vi "LDA_IP.vi"() -> (15 "error out":errorcluster)   [LabVIEW 2012]
uses:
  Globals/Meas_global.vi
  Globals/LDA_meas_global_1.vi
  Globals/LDA_meas_global_2.vi
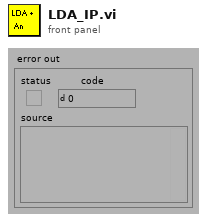
[diagram p1: front panel]
types:
  T1 = typedef "Ch_and_Spans.ctl" = cluster{"high limit (10V)":sgl, "low limit (-10V)":sgl, "Ch No":i16, "Var name":string, "Use Latest Calib":bool}
  T2 = typedef "LDA_Setup.ctl" = cluster{"dimensions":enum16{"1D", "2D"}, "Analogue Freq Multiplier":dbl}
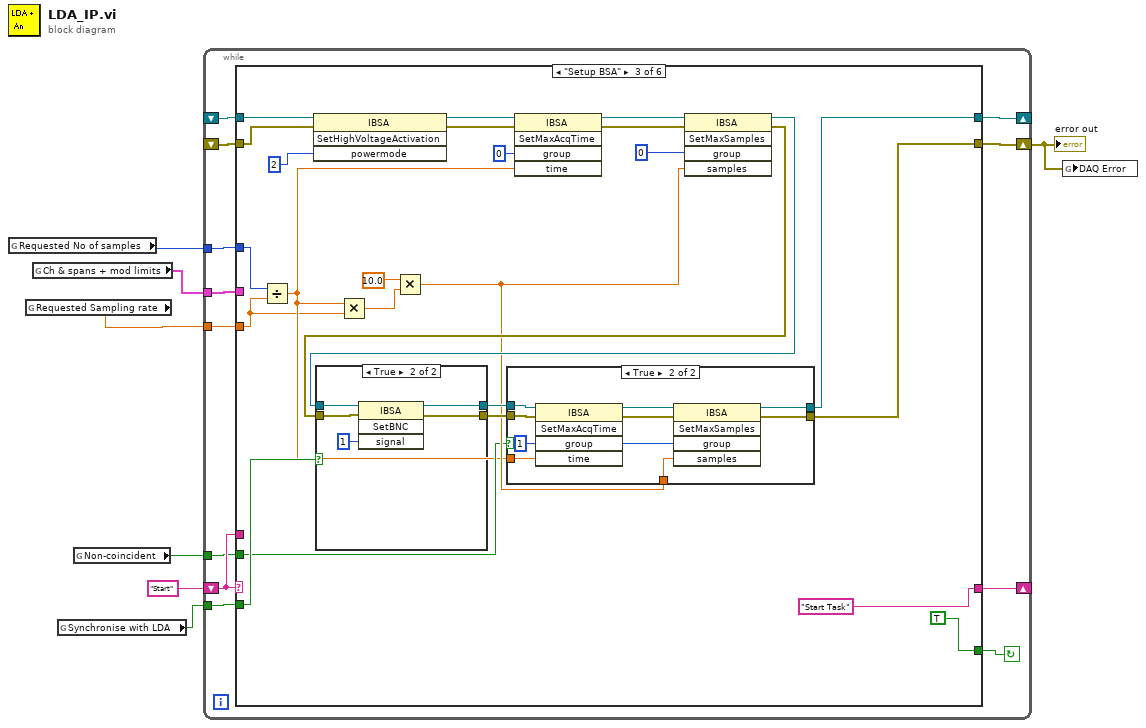
[diagram p0: block diagram]
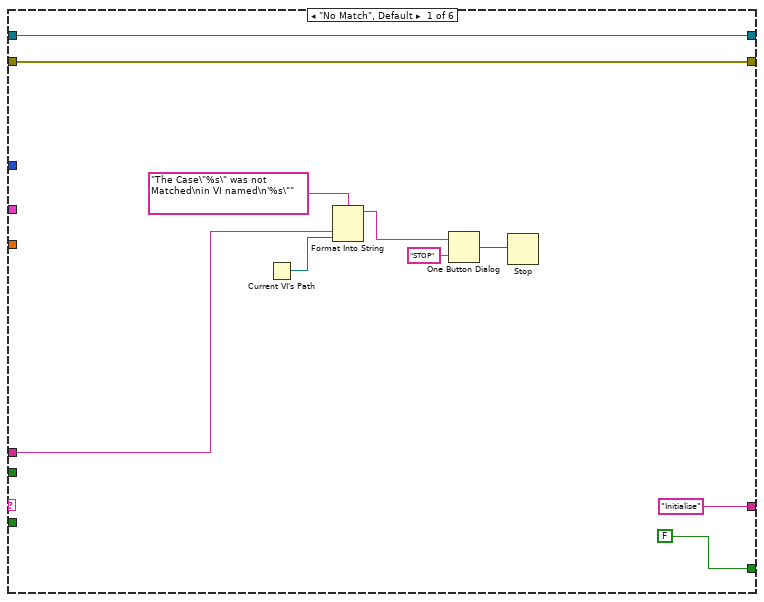
[diagram p2: hidden frame]
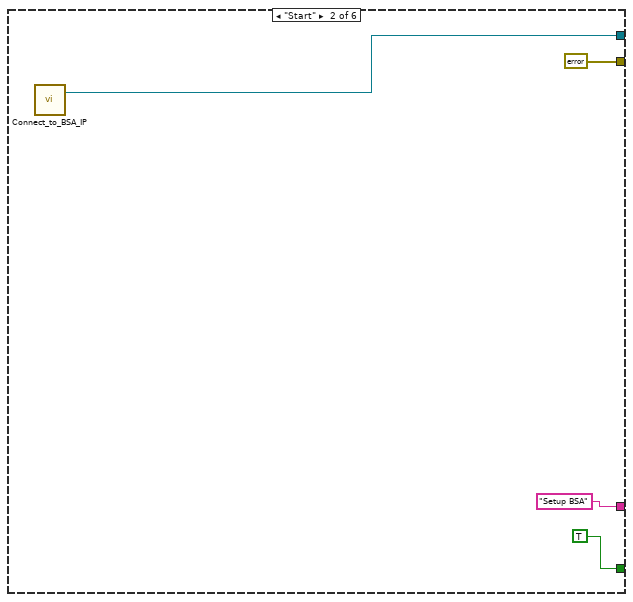
[diagram p3: hidden frame]
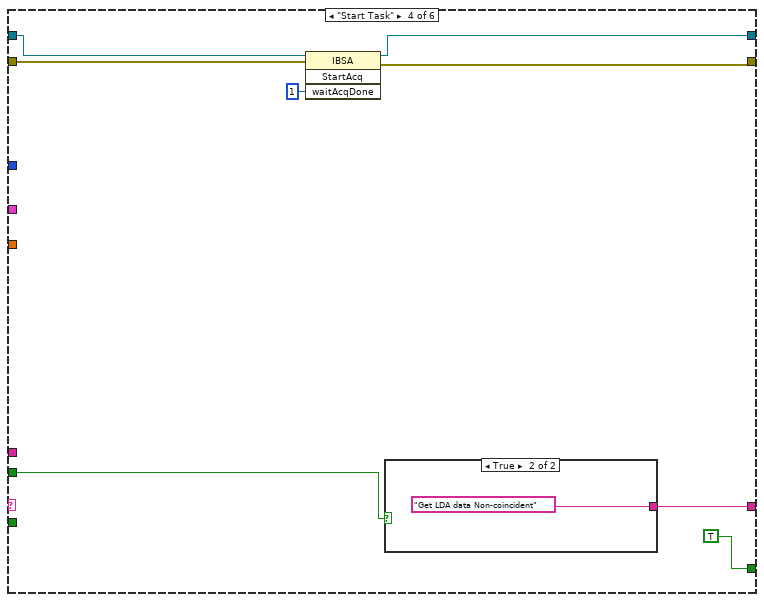
[diagram p6: hidden frame]
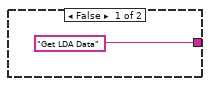
[diagram p7: hidden frame]
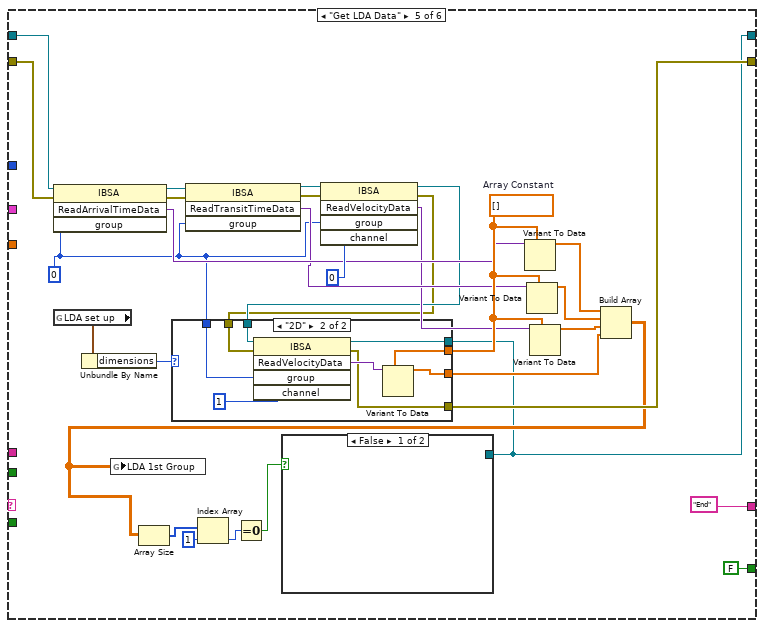
[diagram p8: hidden frame]
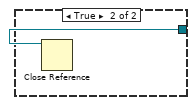
[diagram p9: hidden frame]
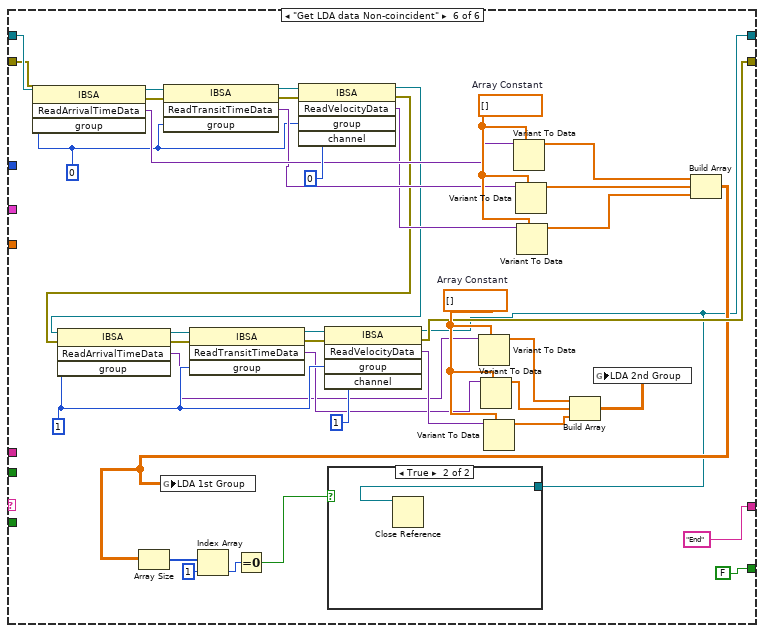
[diagram p11: hidden frame]
diagram:
  n1 = global read "Meas_global.vi" "Requested No of samples"() -> (w2:i32)
  n2 = global read "Meas_global.vi" "Requested Sampling rate"() -> (w3:dbl)
  n3 = global read "Meas_global.vi" "Ch & spans + mod limits"() -> (w4:T1[])
  n4 = global read "Meas_global.vi" "Synchronise with LDA"() -> (w6:bool)
  n5 = global read "LDA_meas_global_1.vi" "Non-coincident"() -> (w5:bool)
  n6 = while {
    shift-left: "Start" -> [w17]
    shift-right: [w18] -> _
    shift-right: [w13] -> w1
    shift-left: _ -> [w16]
    tunnel: w2 -> [w15]
    tunnel: w4 -> [w14]
    tunnel: w3 -> [w12]
    shift-right: [w10] -> _
    shift-left: _ -> [w11]
    tunnel: w6 -> [w9]
    tunnel: w5 -> [w8]
    stop <- w19 continue-if-true
    n7 = case shown="\"Setup BSA\"" w17 {
      tunnel: [FALSE TRUE TRUE TRUE FALSE FALSE] -> w19
      tunnel: ["Initialise" "Setup BSA" "Start Task" w79 "End" "End"] -> w18
      tunnel: w17 -> [w24 _ _ _ _ _]
      tunnel: [w21 errorcluster {"status"=FALSE, "code"=0, "source"=""} ("error out") w40 w83 w98 w139] -> w13
      tunnel: w16 -> [w21 _ w49 w80 w92 w137]
      tunnel: w15 -> [_ _ w50 _ _ _]
      tunnel: w14 -> [_ _ _ _ _ _]
      tunnel: w12 -> [_ _ w35 _ _ _]
      tunnel: w11 -> [w20 _ w51 w82 w102 w138]
      tunnel: [w20 w30 w42 w81 w88 w130] -> w10
      tunnel: w9 -> [_ _ w44 _ _ _]
      tunnel: w8 -> [_ _ w38 w78 _ _]
      frame "No Match", Default {
        n8 = Current VI's Path() -> (path=w23:path)
        n9 = Format Into String(format string="The Case\"%s\" was not Matched\nin VI named\n'%s\"" ("Format String"), w24, w23) -> (resulting string=w27:string)  [unwired: 2 in, 1 out]
        n10 = One Button Dialog(message=w27, button name ("OK")="STOP") -> (true=w25:bool)
        n11 = Stop(stop? (T)=w25) -> ()
      }
      frame "Start" {
        n12 = call "Connect_to_BSA_IP.vi"() -> ("BSA"=w30:refnum<k7>)  [unwired: 3 out]
      }
      frame "Setup BSA" {
        n13 = Divide(x=w50, y=w35) -> (x/y=w36:dbl)
        n14 = invoke class="IBSA" method="SetHighVoltageActivation"(reference=w51, error in=w49, "powermode"=2) -> (reference out=w56:refnum<k7>, error out=w58:errorcluster)  [unwired: 1 in, 2 out]
        n15 = Multiply(x=w36, y=w35) -> (x*y=w34:dbl)
        n16 = Multiply(x=10.0 ("y"), y=w34) -> (x*y=w39:dbl)
        n17 = invoke class="IBSA" method="SetMaxAcqTime"(reference=w56, error in=w58, "group"=0, "time"=w36) -> (reference out=w57:refnum<k7>, error out=w55:errorcluster)  [unwired: 1 in, 3 out]
        n18 = invoke class="IBSA" method="SetMaxSamples"(reference=w57, error in=w55, "group"=0, "samples"=w39) -> (reference out=w46:refnum<k7>, error out=w45:errorcluster)  [unwired: 1 in, 3 out]
        n19 = case shown="True" w44 {
          tunnel: w46 -> [w70 w75]
          tunnel: w45 -> [w71 w74]
          tunnel: [w70 w73] -> w43
          tunnel: [w71 w72] -> w41
          frame False {
          }
          frame True {
            n20 = invoke class="IBSA" method="SetBNC"(reference=w75, error in=w74, "signal"=1) -> (reference out=w73:refnum<k7>, error out=w72:errorcluster)  [unwired: 1 in, 2 out]
          }
        }
        n21 = case shown="True" w38 {
          tunnel: w43 -> [w60 w67]
          tunnel: [w60 w65] -> w42
          tunnel: w41 -> [w59 w64]
          tunnel: [w59 w63] -> w40
          tunnel: w36 -> [_ w62]
          tunnel: w39 -> [_ w61]
          frame False {
          }
          frame True {
            w68 = 1 ("group")
            n22 = invoke class="IBSA" method="SetMaxAcqTime"(reference=w67, error in=w64, "group"=w68, "time"=w62) -> (reference out=w66:refnum<k7>, error out=w69:errorcluster)  [unwired: 1 in, 3 out]
            n23 = invoke class="IBSA" method="SetMaxSamples"(reference=w66, error in=w69, "group"=w68, "samples"=w61) -> (reference out=w65:refnum<k7>, error out=w63:errorcluster)  [unwired: 1 in, 3 out]
          }
        }
      }
      frame "Start Task" {
        n24 = invoke class="IBSA" method="StartAcq"(reference=w82, error in=w80, "waitAcqDone"=1) -> (reference out=w81:refnum<k7>, error out=w83:errorcluster)  [unwired: 1 in, 2 out]
        n25 = case shown="True" w78 {
          tunnel: ["Get LDA Data" "Get LDA data Non-coincident"] -> w79
          frame False {
          }
          frame True {
          }
        }
      }
      frame "Get LDA Data" {
        w110 = dbl[] []  # Array Constant
        w99 = 0 ("group")
        n26 = invoke class="IBSA" method="ReadArrivalTimeData"(reference=w102, error in=w92, "group"=w99) -> (reference out=w115:refnum<k7>, error out=w114:errorcluster, "ReadArrivalTimeData"=w109:variant)  [unwired: 1 in, 1 out]
        n27 = global read "Meas_global.vi" "LDA set up"() -> (w91:T2)
        n28 = Unbundle By Name(w91) -> ("dimensions"=w90:enum16{"1D", "2D"})
        n29 = invoke class="IBSA" method="ReadTransitTimeData"(reference=w115, error in=w114, "group"=w99) -> (reference out=w113:refnum<k7>, error out=w112:errorcluster, "ReadTransitTimeData"=w108:variant)  [unwired: 1 in, 1 out]
        n30 = invoke class="IBSA" method="ReadVelocityData"(reference=w113, error in=w112, "group"=w99, "channel"=0) -> (reference out=w101:refnum<k7>, error out=w100:errorcluster, "ReadVelocityData"=w107:variant)  [unwired: 1 in, 2 out]
        n31 = case shown="\"2D\"" w90 {
          tunnel: w110 -> [w118 w127]
          tunnel: [w118 w125] -> w103
          tunnel: [w119 w124] -> w88
          tunnel: w101 -> [w119 w123]
          tunnel: w100 -> [w117 w122]
          tunnel: w99 -> [_ w121]
          tunnel: [w117 w120] -> w98
          frame "1D" {
          }
          frame "2D" {
            n32 = invoke class="IBSA" method="ReadVelocityData"(reference=w123, error in=w122, "group"=w121, "channel"=1) -> (reference out=w124:refnum<k7>, error out=w120:errorcluster, "ReadVelocityData"=w126:variant)  [unwired: 1 in, 2 out]
            n33 = Variant To Data(type=w127, Variant=w126) -> (data=w125:dbl[])  [unwired: 1 in, 1 out]
          }
        }
        n34 = Variant To Data(type=w110, Variant=w109) -> (data=w106:dbl[])  [unwired: 1 in, 1 out]
        n35 = Variant To Data(type=w110, Variant=w108) -> (data=w105:dbl[])  [unwired: 1 in, 1 out]
        n36 = Variant To Data(type=w110, Variant=w107) -> (data=w104:dbl[])  [unwired: 1 in, 1 out]
        n37 = Build Array(w106, w105, w104, w103) -> (w93:dbl[][])
        n38 = global write "LDA_meas_global_2.vi" "LDA 1st Group"(w93) -> ()
        n39 = Array Size(array=w93) -> (size(s)=w97:i32[])
        n40 = Index Array(array=w97, index=1) -> (element=w95:i32)
        n41 = Equal To 0?(x=w95) -> (x = 0?=w94:bool)
        n42 = case shown="False" w94 {
          tunnel: w88 -> [_ w116]
          frame False {
          }
          frame True {
            n43 = Close Reference(reference=w116) -> ()  [unwired: 1 in, 1 out]
          }
        }
      }
      frame "Get LDA data Non-coincident" {
        w146 = dbl[] []  # Array Constant
        w153 = 1 ("group")
        w160 = dbl[] []  # Array Constant
        w154 = 0 ("group")
        n44 = invoke class="IBSA" method="ReadArrivalTimeData"(reference=w138, error in=w137, "group"=w154) -> (reference out=w165:refnum<k7>, error out=w164:errorcluster, "ReadArrivalTimeData"=w159:variant)  [unwired: 1 in, 1 out]
        n45 = invoke class="IBSA" method="ReadTransitTimeData"(reference=w165, error in=w164, "group"=w154) -> (reference out=w163:refnum<k7>, error out=w162:errorcluster, "ReadTransitTimeData"=w158:variant)  [unwired: 1 in, 1 out]
        n46 = invoke class="IBSA" method="ReadVelocityData"(reference=w163, error in=w162, "group"=w154, "channel"=0) -> (reference out=w140:refnum<k7>, error out=w141:errorcluster, "ReadVelocityData"=w157:variant)  [unwired: 1 in, 2 out]
        n47 = invoke class="IBSA" method="ReadArrivalTimeData"(reference=w140, error in=w141, "group"=w153) -> (reference out=w148:refnum<k7>, error out=w149:errorcluster, "ReadArrivalTimeData"=w142:variant)  [unwired: 1 in, 1 out]
        n48 = invoke class="IBSA" method="ReadTransitTimeData"(reference=w148, error in=w149, "group"=w153) -> (reference out=w150:refnum<k7>, error out=w151:errorcluster, "ReadTransitTimeData"=w143:variant)  [unwired: 1 in, 1 out]
        n49 = invoke class="IBSA" method="ReadVelocityData"(reference=w150, error in=w151, "group"=w153, "channel"=1) -> (reference out=w130:refnum<k7>, error out=w139:errorcluster, "ReadVelocityData"=w144:variant)  [unwired: 1 in, 2 out]
        n50 = Variant To Data(type=w146, Variant=w142) -> (data=w147:dbl[])  [unwired: 1 in, 1 out]
        n51 = Variant To Data(type=w146, Variant=w143) -> (data=w145:dbl[])  [unwired: 1 in, 1 out]
        n52 = Variant To Data(type=w146, Variant=w144) -> (data=w134:dbl[])  [unwired: 1 in, 1 out]
        n53 = Variant To Data(type=w160, Variant=w159) -> (data=w156:dbl[])  [unwired: 1 in, 1 out]
        n54 = Variant To Data(type=w160, Variant=w158) -> (data=w155:dbl[])  [unwired: 1 in, 1 out]
        n55 = Variant To Data(type=w160, Variant=w157) -> (data=w135:dbl[])  [unwired: 1 in, 1 out]
        n56 = Build Array(w147, w145, w134) -> (w136:dbl[][])
        n57 = global write "LDA_meas_global_2.vi" "LDA 2nd Group"(w136) -> ()
        n58 = Build Array(w156, w155, w135) -> (w133:dbl[][])
        n59 = Array Size(array=w133) -> (size(s)=w168:i32[])
        n60 = global write "LDA_meas_global_2.vi" "LDA 1st Group"(w133) -> ()
        n61 = Index Array(array=w168, index=1) -> (element=w166:i32)
        n62 = Equal To 0?(x=w166) -> (x = 0?=w132:bool)
        n63 = case shown="True" w132 {
          tunnel: w130 -> [_ w169]
          frame False {
          }
          frame True {
            n64 = Close Reference(reference=w169) -> ()  [unwired: 1 in, 1 out]
          }
        }
      }
    }
  }
  "error out" <- w1
  n65 = global write "Meas_global.vi" "DAQ Error"(w1) -> ()
